vi "TEST.vi"() -> ()   [LabVIEW 2020]
panel:
  out "error out":errorcluster
  out "read buffer":string
  in  "VISA resource name":refnum<visa-resource-name>
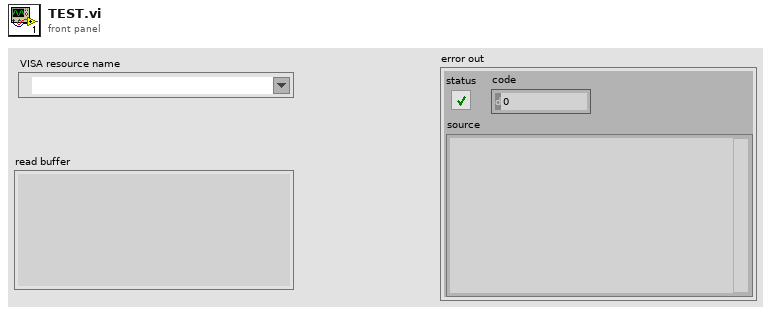
[diagram p1: front panel]
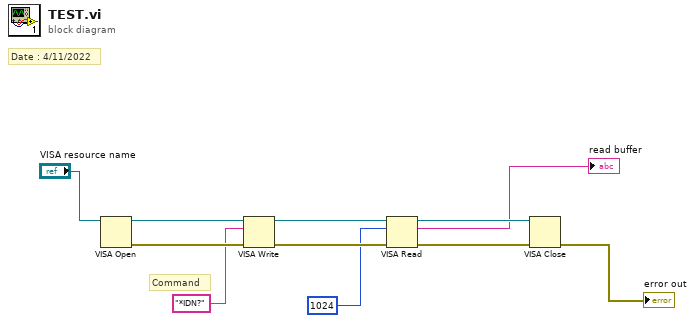
[diagram p0: block diagram]
diagram:
  # "Date : 4/11/2022"
  # "Command"
  n1 = VISA Open(VISA resource name="VISA resource name") -> (VISA resource name=w11:refnum<visa-resource-name>, error out=w8:errorcluster)  [unwired: 4 in]
  n2 = VISA Write(VISA resource name=w11, write buffer="*IDN?", error in (no error)=w8) -> (VISA resource name out=w10:refnum<visa-resource-name>, error out=w7:errorcluster)  [unwired: 1 out]
  n3 = VISA Read(VISA resource name=w10, byte count=u32 1024, error in (no error)=w7) -> (VISA resource name out=w9:refnum<visa-resource-name>, read buffer=→"read buffer":string, error out=w6:errorcluster)  [unwired: 1 out]
  n4 = VISA Close(VISA resource name=w9, error in (no error)=w6) -> (error out=→"error out":errorcluster)
